vi "DefineNetCDFFileName.vi"(8 "ErrorIn":errorcluster, 10 "WVDialNumber":dbl=2.0, 11 "BasePath":string) -> (0 "ErrorOut":errorcluster, 2 "BaseName":string, 3 "FullFileName":string="TestingNCARWVDIAL002.20171024_085111.cdf")   [LabVIEW 2012]
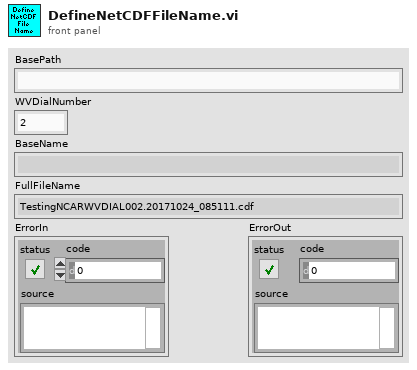
[diagram p1: front panel]
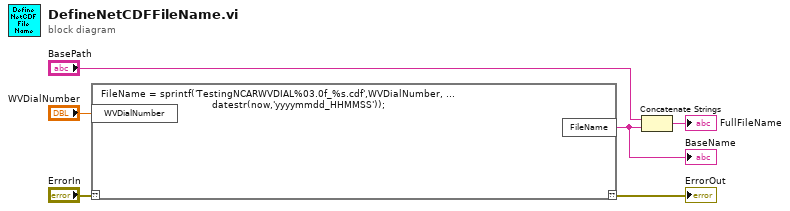
[diagram p0: block diagram]
diagram:
  n1 = script code="FileName = sprintf('TestingNCARWVDIAL%03.0f_%s.cdf',WVDialNumber, ...\n                                     datestr(now,'yyyymmdd_HHMMSS'));"("??"="ErrorIn", "WVDialNumber"="WVDialNumber") -> ("??"=→"ErrorOut":errorcluster, "FileName"=w2:string)
  "BaseName" <- w2
  n2 = Concatenate Strings("BasePath", w2) -> (→"FullFileName":string)
